vi "TC_to_DSC.vi"(7 "Enum":enum16{"CF", "MNK", "MNK_Z_Bridge"}(ring)=enum."MNK", 9 "I":dbl[](array[numeric]), 10 "T":dbl[](array[numeric]), 11 "R":dbl[](array[numeric])) -> ()   [LabVIEW 2013]
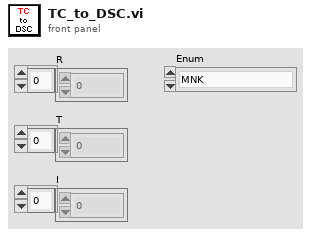
[diagram p1: front panel]
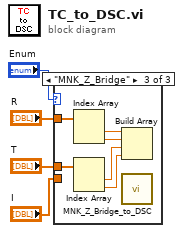
[diagram p0: block diagram]
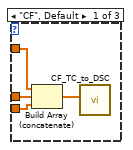
[diagram p2: hidden frame]
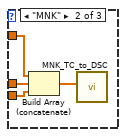
[diagram p3: hidden frame]
diagram:
  n1 = case shown="\"MNK_Z_Bridge\"" "Enum" {
    tunnel: "R" -> [w8 w12 w17]
    tunnel: "T" -> [w7 w11 w18]
    tunnel: "I" -> [w6 w10 _]
    frame "CF", Default {
      n2 = Build Array (concatenate)(w8, w7, w6) -> (w5:dbl[])
      n3 = call "CF_TC_to_DSC.vi"("dbl"=w5) -> ()  [unwired: 3 in]
    }
    frame "MNK" {
      n4 = Build Array (concatenate)(w12, w11, w10) -> (w9:dbl[])
      n5 = call "MNK_TC_to_DSC.vi"("dbl"=w9) -> ()  [unwired: 3 in]
    }
    frame "MNK_Z_Bridge" {
      n6 = Index Array(array=w17) -> (element #1=w16:dbl, element #2=w15:dbl)  [unwired: 2 in]
      n7 = Index Array(array=w18) -> (element #1=w14:dbl, element #2=w13:dbl)  [unwired: 2 in]
      n8 = Build Array(w16, w15, w14, w13) -> ()  [unwired: 1 out]
      n9 = call "MNK_Z_Bridge_to_DSC.vi"() -> ()  [unwired: 4 in]
    }
  }
